vi "(SUBTASK 1&2) - Follow line.vi"() -> ()   [LabVIEW 2016, in "testrobot.lvrbt"]
uses:
  testrobot.lvrbt
  <vilib>/NXT/Subs/LVHSConnector.ctl
  <vilib>/NXT/LegoClasses/BrickReference/BrickReference.lvclass
  <vilib>/NXT/Block Support/NXT_InputPort.ctl
panel:
  out "NXT/EV3 2":T1
  in  "Left Light \nSensor":T2 items=["Port 1", "Port 2", "Port 3", "Port 4"]
  in  "Right Light\n Sensor":T2=3 items=["Port 1", "Port 2", "Port 3", "Port 4"]
  out "only right":bool
  out "both negative":bool
  out "Go Straight":bool
  out "Turn Left":bool
  out "Turn Right":bool
  out "Display\nRight Light\nSensor":sgl
  out "Display\nLeft Light\nSensor":sgl
  in  "NXT/EV3":T1
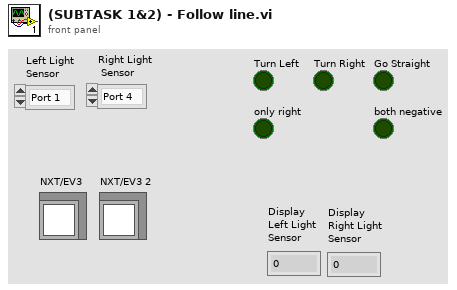
[diagram p1: front panel]
types:
  T1 = typedef "LVHSConnector.ctl" = refnum<class "BrickReference.lvclass">
  T2 = typedef "NXT_InputPort.ctl" = u32
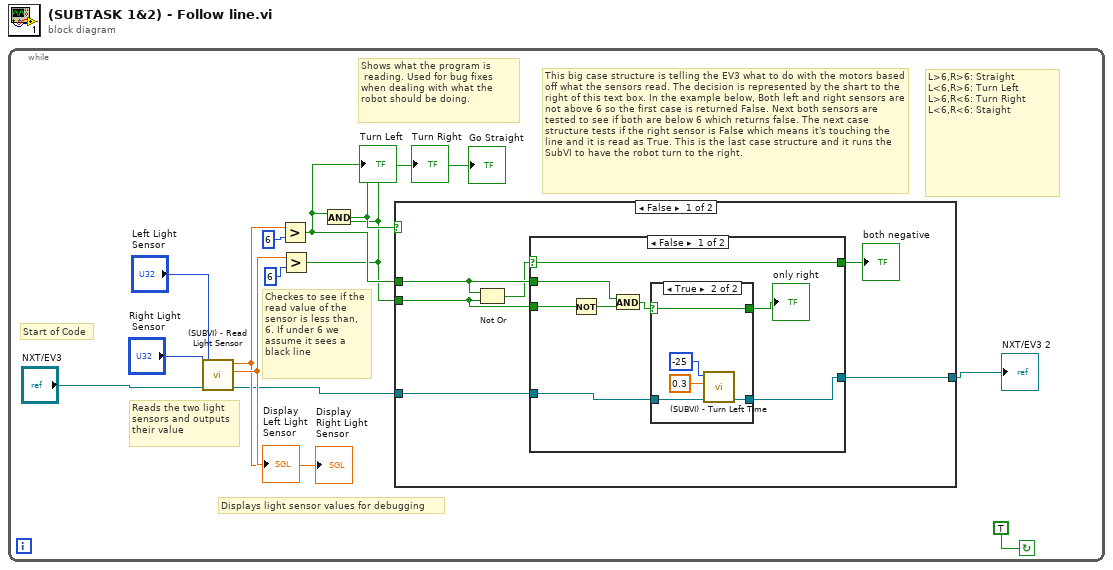
[diagram p0: block diagram]
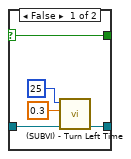
[diagram p2: hidden frame]
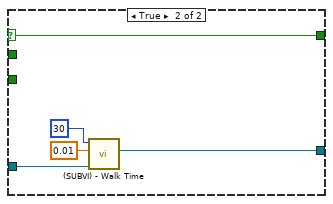
[diagram p3: hidden frame]
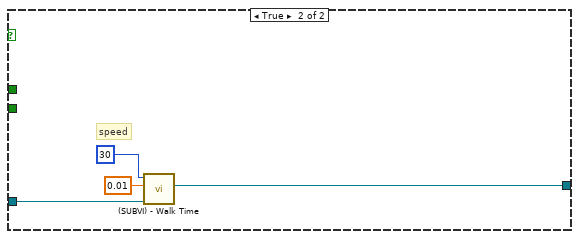
[diagram p4: hidden frame]
diagram:
  n1 = while {
    stop <- TRUE continue-if-true
    # "L>6,R>6: Straight\nL<6,R>6: Turn Left \nL>6,R<6: Turn Right\nL<6,R<6: Staight"
    # "This big case structure is telling the EV3 what to do with the motors based off what the sensors read. The decision is represented by the shart to the right of this text box. In the example below, Both left and right sensors are not above 6 so the first case is returned False. Next both sensors are tested to see if both are below 6 which returns false. The next case structure tests if the right sensor is False which means it's touching the line and it is read as True. This is the last case structure and it runs the SubVI to have the robot turn to the right."
    # "Displays light sensor values for debugging"
    # "Checkes to see if the read value of the sensor is less than, 6. If under 6 we assume it sees a black line"
    # "Shows what the program is\n reading. Used for bug fixes when dealing with what the robot should be doing."
    # "Reads the two light\nsensors and outputs\ntheir value"
    # "Start of Code"
    n2 = call "(SUBVI) - Read Light Sensor.vi"("NXT/EV3"="NXT/EV3", "Port (Port 1) 2"="Right Light\n Sensor", "Port (Port 1)"="Left Light \nSensor") -> ("NXT/EV3 2"=w8:T1, "Scaled Value 2"=w11:sgl, "Scaled Value"=w10:sgl)  [unwired: 6 in]
    "Display\nLeft Light\nSensor" <- w11
    "Display\nRight Light\nSensor" <- w10
    n3 = Greater?(x=w10, y=6) -> (0:w7:bool)
    "Turn Right" <- w7
    n4 = Greater?(x=w11, y=6) -> (0:w6:bool)
    "Turn Left" <- w6
    n5 = And(x=w7, y=w6) -> (x .and. y?=w9:bool)
    "Go Straight" <- w9
    n6 = case shown="False" w9 {
      tunnel: w8 -> [w15 w44]
      tunnel: [w14 w43] -> w2
      tunnel: w7 -> [w18 _]
      tunnel: w6 -> [w17 _]
      frame False {
        n7 = Not Or(1:w17, 2:w18) -> (0:w16:bool)
        n8 = case shown="False" w16 {
          selector: w16 -> [w27 w42]
          tunnel: [w27 w42] -> w19
          tunnel: w18 -> [w25 _]
          tunnel: w17 -> [w23 _]
          tunnel: w15 -> [w21 w39]
          tunnel: [w20 w38] -> w14
          frame False {
            n9 = Not(x=w23) -> (.not. x?=w24:bool)
            n10 = And(x=w25, y=w24) -> (x .and. y?=w26:bool)
            n11 = case shown="True" w26 {
              selector: w26 -> [w32 w37]
              tunnel: [w32 w37] -> w22
              tunnel: w21 -> [w29 w34]
              tunnel: [w28 w33] -> w20
              frame False {
                n12 = call "(SUBVI) - Turn Left Time.vi"("NXT/EV3"=w29, "Time walking"=0.3, "Walk Speed"=25) -> ("NXT/EV3 2"=w28:T1)  [unwired: 8 in]
              }
              frame True {
                n13 = call "(SUBVI) - Turn Left Time.vi"("NXT/EV3"=w34, "Time walking"=0.3, "Walk Speed"=-25) -> ("NXT/EV3 2"=w33:T1)  [unwired: 8 in]
              }
            }
            "only right" <- w22
          }
          frame True {
            n14 = call "(SUBVI) - Walk Time.vi"("NXT/EV3"=w39, "Time walking"=0.01, "Walk Speed"=30) -> ("NXT/EV3 2"=w38:T1)  [unwired: 8 in]
          }
        }
        "both negative" <- w19
      }
      frame True {
        # "speed"
        n15 = call "(SUBVI) - Walk Time.vi"("NXT/EV3"=w44, "Time walking"=0.01, "Walk Speed"=30) -> ("NXT/EV3 2"=w43:T1)  [unwired: 8 in]
      }
    }
    "NXT/EV3 2" <- w2
  }
